vi "unixToStrTime.vi"(11 "unix time":dbl) -> (3 "date/time string":string)   [LabVIEW 2016]
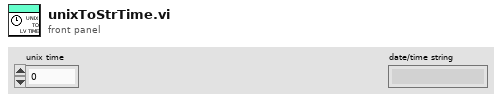
[diagram p1: front panel]
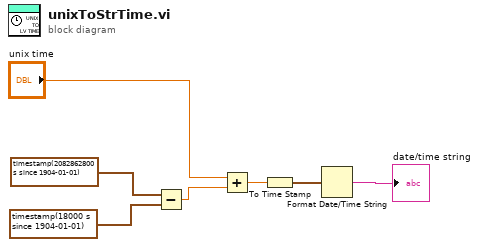
[diagram p0: block diagram]
diagram:
  n1 = Subtract(x=timestamp(2082862800 s since 1904-01-01), y=timestamp(18000 s since 1904-01-01)) -> (x-y=w5:dbl)
  n2 = Add(x="unix time", y=w5) -> (x+y=w3:dbl)
  n3 = To Time Stamp(1:w3) -> (0:w2:timestamp)
  n4 = Format Date/Time String(seconds (now)=w2) -> (date/time string=→"date/time string":string)  [unwired: 2 in]
